vi "MiliVolt2Level.vi"(1 "voltage /V":dbl) -> (0 "level":i16)   [LabVIEW 2017]
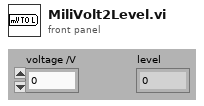
[diagram p1: front panel]
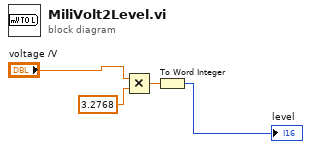
[diagram p0: block diagram]
diagram:
  n1 = Multiply(x="voltage /V", y=3.2768) -> (x*y=w3:dbl)
  n2 = To Word Integer(number=w3) -> (16bit integer=→"level":i16)
